vi "Designate Abstract Method.vi"(8 "error in (no error)":errorcluster, 11 "LabVIEW Object in":refnum<class>) -> (0 "error out":errorcluster, 3 "LabVIEW Object out":refnum<class>)   [LabVIEW 2020, in "Utilities.lvlib"]
doc: "Helpful for designating a method as an abstract method. This VI will generate an error if the VI containing it is called."
uses:
  Utilities.lvlib
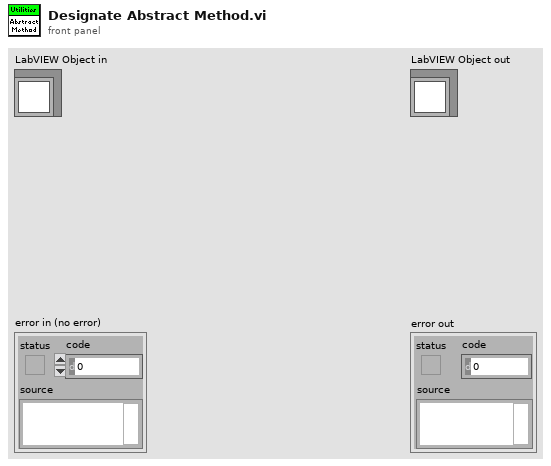
[diagram p1: front panel]
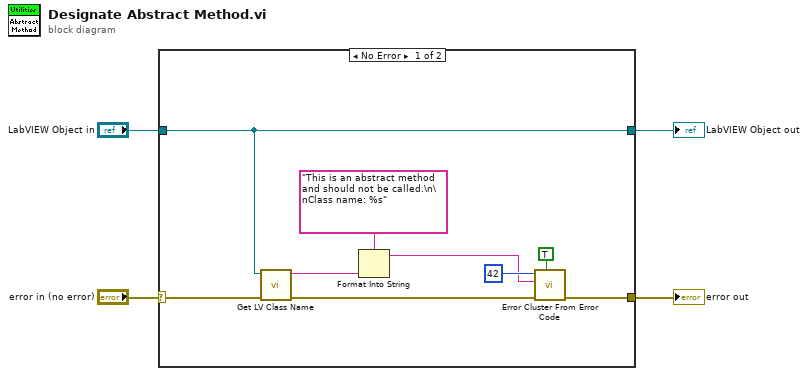
[diagram p0: block diagram]
diagram:
  n1 = case shown="No Error" "error in (no error)" {
    selector: "error in (no error)" -> [w10 w15]
    tunnel: [w11 w15] -> w4
    tunnel: "LabVIEW Object in" -> [w8 w14]
    tunnel: [w8 w14] -> w1
    frame No Error {
      n2 = call <vilib>:"Get LV Class Name.vi"("error in (no error)"=w10, "object"=w8) -> ("error out"=w9:errorcluster, "class name"=w6:string)  [unwired: 8 in]
      n3 = Format Into String(format string="This is an abstract method and should not be called.\n\nClass name: %s", w6) -> (resulting string=w5:string)  [unwired: 2 in, 1 out]
      n4 = call <vilib>:"Error Cluster From Error Code.vi"("show call chain? (False)"=TRUE, "error in (no error)"=w9, "error message (\"\")"=w5, "error code (0)"=42) -> ("error out"=w11:errorcluster)  [unwired: 5 in]
    }
    frame Error {
    }
  }
  "error out" <- w4
  "LabVIEW Object out" <- w1
